vi "Demo Daemon.vi"(10 "Data":string, 11 "Name":string) -> ()   [LabVIEW 2018, in "Thread.lvlib"]
uses:
  Thread.lvlib
panel:
  out "ms Remaining":u32
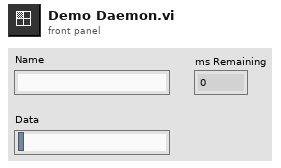
[diagram p1: front panel]
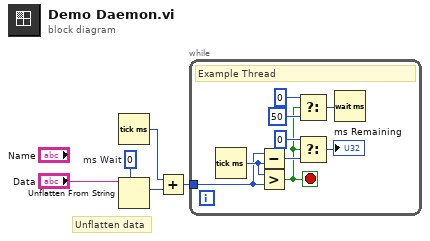
[diagram p0: block diagram]
diagram:
  w5 = u32 0  # ms Wait
  # "Unflatten data"
  n1 = Tick Count (ms)() -> (millisecond timer value=w3:u32)
  n2 = Unflatten From String(type=w5, binary string="Data") -> (value=w2:u32)  [unwired: 3 in, 2 out]
  n3 = Add(x=w3, y=w2) -> (x+y=w1:u32)
  n4 = while {
    tunnel: w1 -> [w13]
    stop <- w8 stop-if-true
    # "Example Thread"
    n5 = Tick Count (ms)() -> (millisecond timer value=w14:u32)
    n6 = Subtract(x=w13, y=w14) -> (x-y=w11:u32)
    n7 = Greater?(x=w14, y=w13) -> (0:w8:bool)
    n8 = Select(t=u32 0, s=w8, f=u32 50 ("milliseconds to wait")) -> (s? t:f=w6:u32)
    n9 = Select(t=u32 0, s=w8, f=w11) -> (s? t:f=→"ms Remaining":u32)
    n10 = Wait (ms)(milliseconds to wait=w6) -> ()  [unwired: 1 out]
  }
